vi "GE 5565PIORC.Open.vi"() -> (0 "error out":errorcluster, 3 "GE 5565PIORC":refnum<class "GE 5565PIORC.lvclass">)   [LabVIEW 2016]
uses:
  <vilib>/NI/GE Reflective Memory Driver/GE 5565PIORC.lvclass
  <vilib>/NI/GE Reflective Memory Driver/GE 5565PIORC.lvclass/GE 5565PIORC.ctl
  <vilib>/NI/GE Reflective Memory Driver/Properties/Registers/GE 5565PIORC.Registers.LAS1RR.PCI Address Range.Get.vi
  <vilib>/NI/GE Reflective Memory Driver/Properties/Registers/GE 5565PIORC.Registers.Local Configuration.Read.vi
  <vilib>/NI/GE Reflective Memory Driver/Properties/Registers/GE 5565PIORC.Registers.Local Configuration.Read (U32).vi
  <vilib>/NI/GE Reflective Memory Driver/Methods/GE 5565PIORC.Registers.Read.vi
  <vilib>/NI/GE Reflective Memory Driver/Methods/GE 5565PIORC.Registers.Read (U32).vi
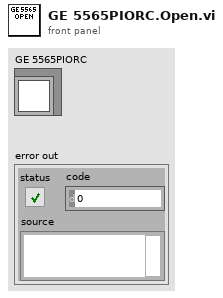
[diagram p1: front panel]
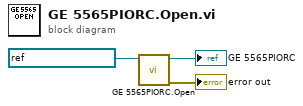
[diagram p0: block diagram]
diagram:
  n1 = call <vilib>:"GE 5565PIORC.Open.vi"("VISA resource name"=refnum<visa-resource-name> "PXI4::14::INSTR") -> ("error out"=→"error out":errorcluster, "GE 5565PIORC.lvclass"=→"GE 5565PIORC":refnum<class "GE 5565PIORC.lvclass">)  [unwired: 9 in]
